vi "Playback Wait.vi"(8 "error in (no error)":errorcluster, 11 "Audio Device Refnum In":T1) -> (0 "error out":errorcluster, 3 "Audio Device Refnum Out":T1)   [LabVIEW 2020, in "G-Audio.lvlib"]
doc: "Wait for the audio device to finish playback of all audio data in its buffer.\n\nWill return an error if used with a capture audio device."
uses:
  G-Audio.lvlib
  Controls/Audio Device Refnum.ctl
  <vilib>/Utility/error.llb/Error Cluster From Error Code.vi
  lib/g_audio_32.dll
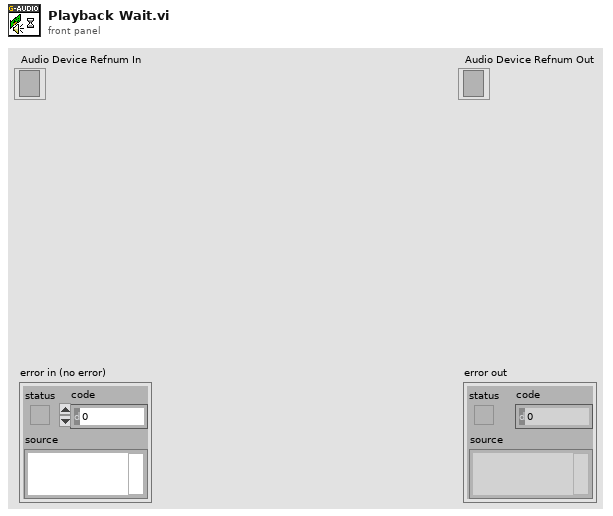
[diagram p1: front panel]
types:
  T1 = typedef "G-Audio.lvlib/Audio Device Refnum.ctl" = refnum<file>
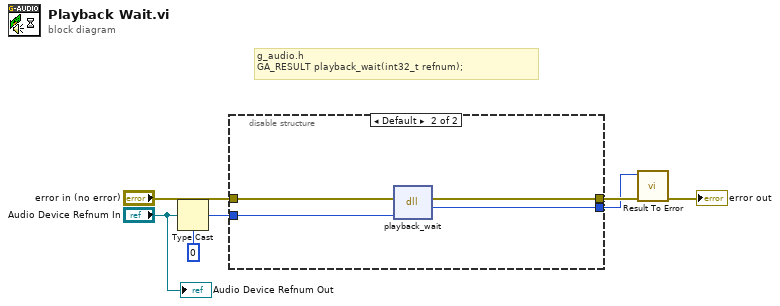
[diagram p0: block diagram]
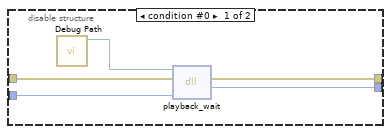
[diagram p2: hidden frame]
diagram:
  # "g_audio.h\nGA_RESULT playback_wait(int32_t refnum);"
  n1 = Type Cast(type=0, x="Audio Device Refnum In") -> (*(type *) &x=w4:i32)
  n2 = disable-structure shown="Default" {
    disable-tunnel: [w11 w16] -> w7
    disable-tunnel: [w10 w15] -> w6
    disable-tunnel: w4 -> [w9 w14]
    disable-tunnel: "error in (no error)" -> [w8 w13]
    frame condition #0 {
      n3 = call "Debug Path.vi"() -> ("Debug Path"=w12:path)  [unwired: 11 in]
      n4 = dll-call lib="?" fn="playback_wait"(path in=w12, error in=w8, "refnum"=w9) -> (error out=w11:errorcluster, "result"=w10:i32)  [unwired: 2 in, 1 out]
    }
    frame condition #1 (active) {
      n5 = dll-call lib="C:/github/dataflowg/g-audio/src/LabVIEW/G-Audio/lib/g_audio_*.*" fn="playback_wait"(error in=w13, "refnum"=w14) -> (error out=w16:errorcluster, "result"=w15:i32)  [unwired: 3 in, 1 out]
    }
  }
  n6 = call "Result To Error.vi"("error in (no error)"=w7, "Result Code"=w6) -> ("error out"=→"error out":errorcluster)  [unwired: 9 in]
  "Audio Device Refnum Out" <- "Audio Device Refnum In"
